vi "Grab Tag Information.vi"(8 "error in":errorcluster, 11 "VI Ref in":refnum<vi>) -> (0 "error out":errorcluster, 1 "Control Info":T1[](array[typedef]) {"tab level" items=["N/A", "FAB--icon--rounded", "outline--icon--rectangular", "outline--icon--rounded", "outline--text--rectangular", "outline--text--rounded", "nooutline--icon--rectangular", "nooutline--icon--rectangular--40x40", "nooutline--icon--rounded", "nooutline--text--rectangular", "nooutline--text--rounded", "tonal--icon--rectangular", "tonal--icon--rounded", "tonal--text--rectangular", "tonal--text--rounded", "filled--icon--rectangular", "filled--icon--rounded", "filled--text--rectangular", "filled--text--rounded"]; "Boolean Type" items=["N/A", "FAB--icon--rounded", "outline--icon--rectangular", "outline--icon--rounded", "outline--text--rectangular", "outline--text--rounded", "nooutline--icon--rectangular", "nooutline--icon--rectangular--40x40", "nooutline--icon--rounded", "nooutline--text--rectangular", "nooutline--text--rounded", "tonal--icon--rectangular", "tonal--icon--rounded", "tonal--text--rectangular", "tonal--text--rounded", "filled--icon--rectangular", "filled--icon--rounded", "filled--text--rectangular", "filled--text--rounded"]; "UI Theme Level" items=["N/A", "Primary", "Secondary", "Tertiary", "Error", "Primary Fixed", "Secondary Fixed", "Tertiary Fixed", "Label Only", "No Change"]}, 2 "map data":map{string, refnum<vi>}(c390), 3 "VI Ref out":refnum<vi>)   [LabVIEW 2021]
doc: "Get the tag data for all the controls on the front panel.\n\n<b>Code Developed By:</b>\nDaniel Coons\nTechnology Service Corporation\nwww.tsc.com/atcs"
uses:
  Material SubVIs/Material SubVIs.lvlib
  control info--typedef.ctl
  <vilib>/Utility/traverseref.llb/TRef TravTarget.ctl
  <vilib>/Utility/traverseref.llb/VI Scripting - Traverse.lvlib
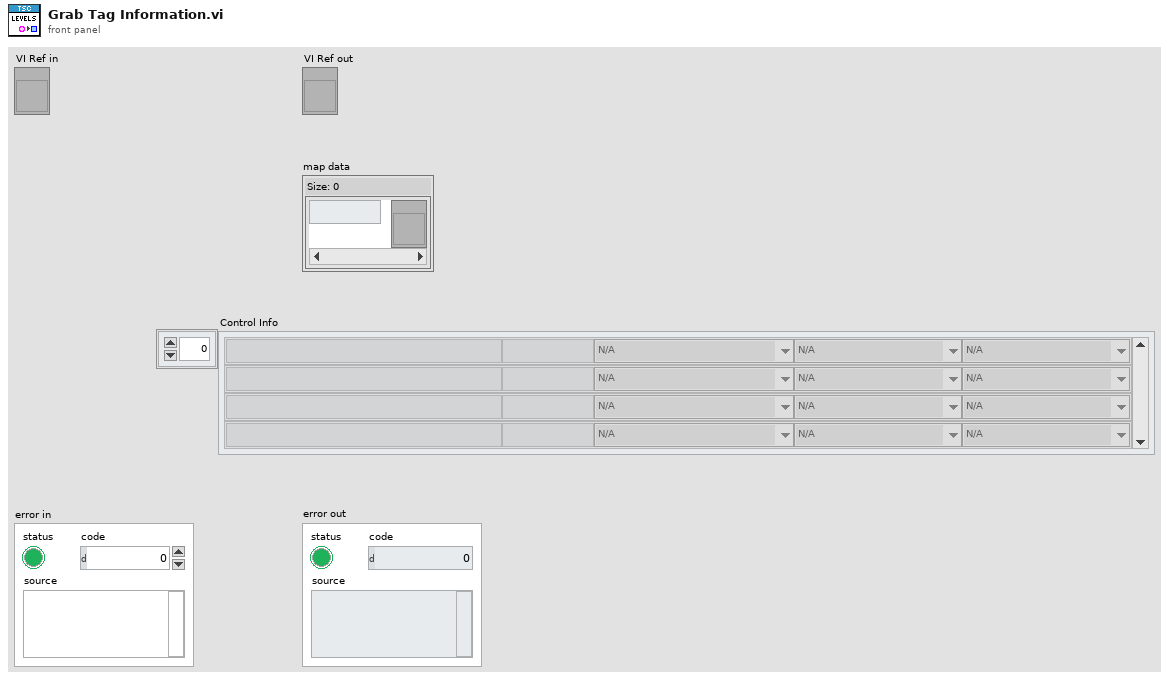
[diagram p1: front panel]
types:
  T1 = typedef "control info--typedef.ctl" = cluster{"label":string, "control type":string, "UI Theme Level":u16, "Boolean Type":u16, "tab level":u16}
  T2 = typedef "TRef TravTarget.ctl" = enum16{"FP", "BD", "Other"}
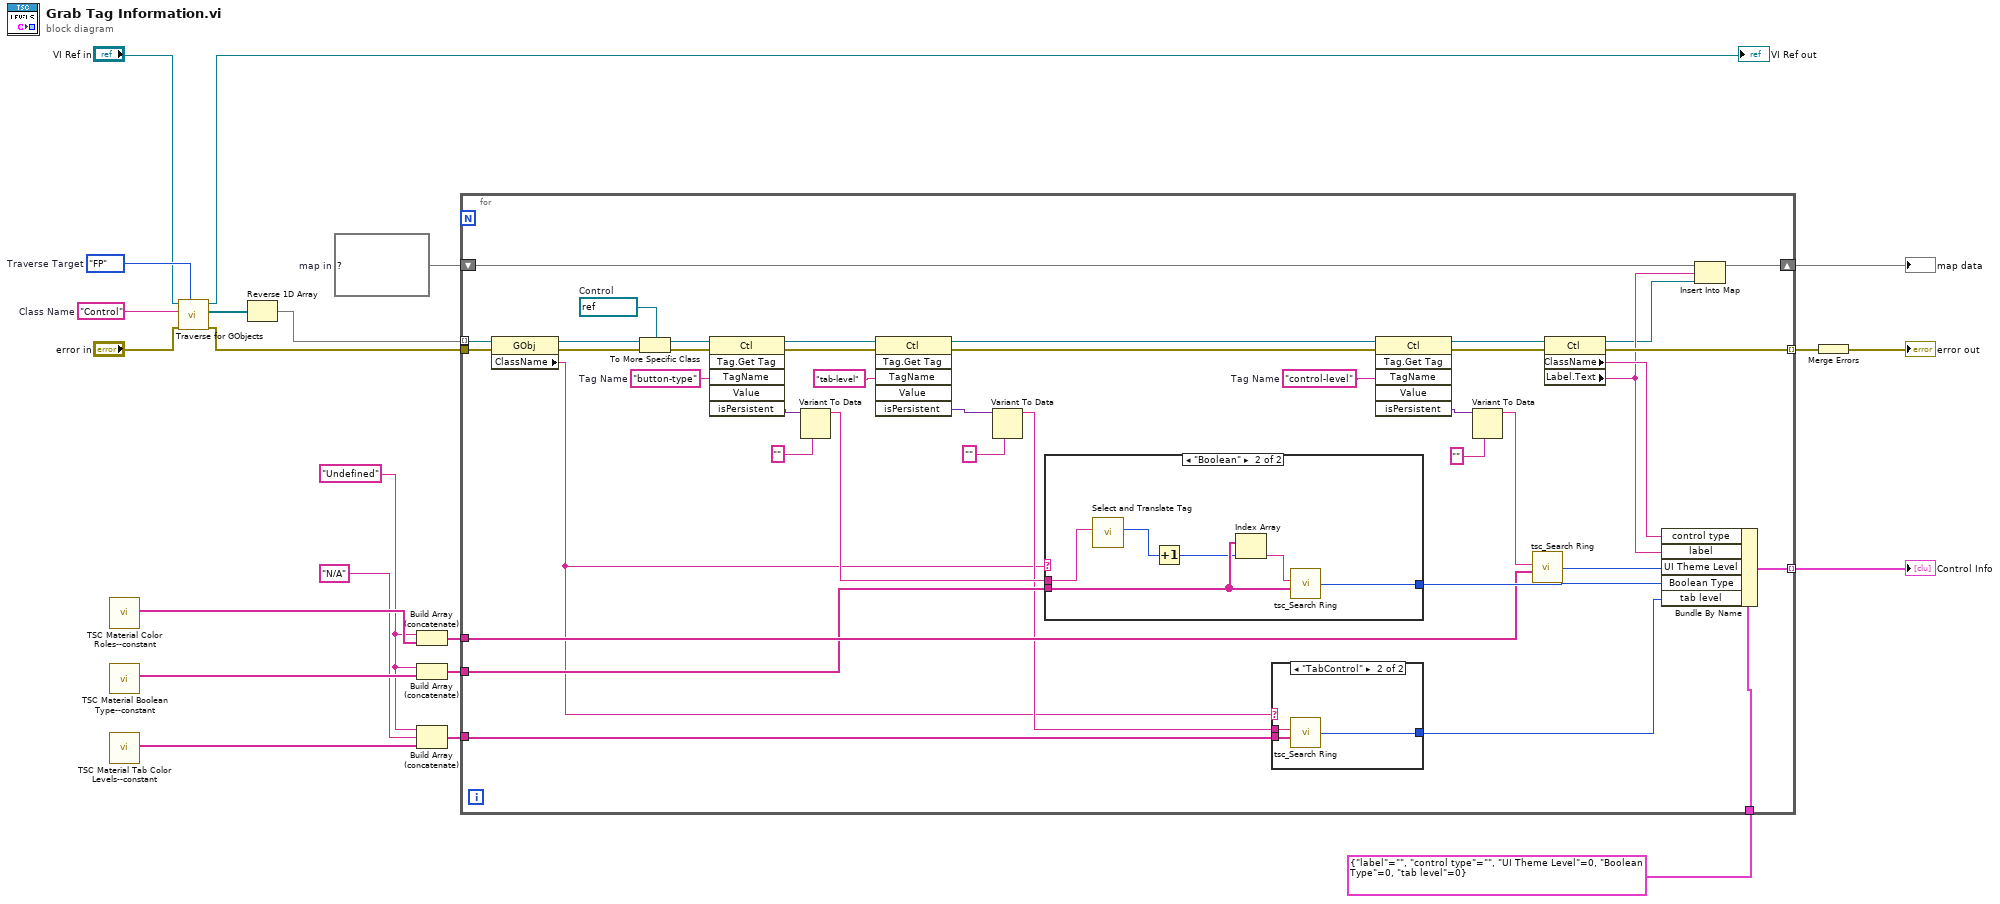
[diagram p0: block diagram]
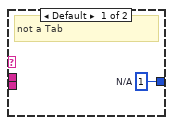
[diagram p2: hidden frame]
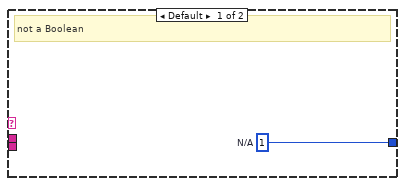
[diagram p3: hidden frame]
diagram:
  w11 = TRef_TravTarget."FP"  # Traverse Target
  w12 = "Control"  # Class Name
  w4 = "Undefined"
  w18 = map{string, refnum<vi>} {}  # map in
  n1 = call "TSC Material Color Roles--constant.vi"() -> ("Control Color Roles"=w15:string[])  [unwired: 11 in]
  n2 = call "TSC Material Boolean Type--constant.vi"() -> ("boolean types"=w5:string[])  [unwired: 11 in]
  n3 = call "TSC Material Tab Color Levels--constant.vi"() -> ("tab color levels"=w2:string[])  [unwired: 11 in]
  n4 = call <vilib>:"Traverse for GObjects.vi"("Traverse Target"=w11, "error in (no error)"="error in", "Class Name"=w12, "VI Refnum"="VI Ref in") -> ("error out"=w21:errorcluster, "References"=w10:refnum<vi>[], "dup VI Refnum"=→"VI Ref out":refnum<vi>)  [unwired: 4 in, 1 out]
  n5 = Reverse 1D Array(array=w10) -> (reversed array=w8:refnum<vi>[])
  n6 = Build Array (concatenate)(w4, w15) -> (w14:string[])
  n7 = Build Array (concatenate)(w4, w5) -> (w13:string[])
  n8 = Build Array (concatenate)(w4, "N/A", w2) -> (w1:string[])
  n9 = for {
    tunnel: w8 -> [w34] mode=indexing
    tunnel: w21 -> [w62]
    tunnel: [w59] -> w7 mode=indexing
    tunnel: T1 {"label"="", "control type"="", "UI Theme Level"=0, "Boolean Type"=0, "tab level"=0} ("control info") -> [w48]
    tunnel: [w46] -> w17 mode=indexing
    shift-right: [w44] -> w19
    shift-left: w18 -> [w45]
    tunnel: w14 -> [w37]
    tunnel: w13 -> [w36]
    tunnel: w1 -> [w24]
    w49 = refnum<vi> refnum  # Control
    w52 = "control-level"  # Tag Name
    w57 = "button-type"  # Tag Name
    n10 = property class="GObj"(reference=w34, error in=w62) -> (reference out=w33:refnum<vi>, error out=w35:errorcluster, "ClassName"=w25:string)
    n11 = To More Specific Class(target class=w49, reference=w33, error in=w35) -> (specific class reference=w50:refnum<vi>, error out=w58:errorcluster)
    n12 = invoke class="Ctl" method="Tag.Get Tag"(reference=w50, error in=w58, "TagName"=w57) -> (reference out=w31:refnum<vi>, error out=w61:errorcluster, "isPersistent"=w56:variant)  [unwired: 3 in, 3 out]
    n13 = Variant To Data(type="", Variant=w56) -> (data=w39:string)  [unwired: 1 in, 1 out]
    n14 = invoke class="Ctl" method="Tag.Get Tag"(reference=w31, error in=w61, "TagName"="tab-level" ("Tag Name")) -> (reference out=w30:refnum<vi>, error out=w32:errorcluster, "isPersistent"=w27:variant)  [unwired: 3 in, 3 out]
    n15 = Variant To Data(type="", Variant=w27) -> (data=w26:string)  [unwired: 1 in, 1 out]
    n16 = case shown="\"Boolean\"" w25 {
      tunnel: w39 -> [_ w72]
      tunnel: [w67 w73] -> w38
      tunnel: w36 -> [_ w70]
      frame Default {
        w67 = u16 1  # N/A
        # "not a Boolean"
      }
      frame "Boolean" {
        n17 = call "Select and Translate Tag.vi"("Current Item"=w72) -> ("index of element"=w71:i32)  [unwired: 10 in]
        n18 = Increment(x=w71) -> (x+1=w68:i32)
        n19 = Index Array(array=w70, index=w68) -> (element=w69:string)
        n20 = call "tsc_Search Ring.vi"("Values"=w70, "Search Item"=w69) -> ("Index"=w73:u16)  [unwired: 2 in]
      }
    }
    n21 = case shown="\"TabControl\"" w25 {
      tunnel: w26 -> [_ w66]
      tunnel: [w63 w65] -> w23
      tunnel: w24 -> [_ w64]
      frame Default {
        w63 = u16 1  # N/A
        # "not a Tab"
      }
      frame "TabControl" {
        n22 = call "tsc_Search Ring.vi"("Values"=w64, "Search Item"=w66) -> ("Index"=w65:u16)  [unwired: 2 in]
      }
    }
    n23 = invoke class="Ctl" method="Tag.Get Tag"(reference=w30, error in=w32, "TagName"=w52) -> (reference out=w51:refnum<vi>, error out=w60:errorcluster, "isPersistent"=w53:variant)  [unwired: 3 in, 3 out]
    n24 = Variant To Data(type="", Variant=w53) -> (data=w41:string)  [unwired: 1 in, 1 out]
    n25 = call "tsc_Search Ring.vi"("Values"=w37, "Search Item"=w41) -> ("Index"=w40:u16)  [unwired: 2 in]
    n26 = property class="Ctl"(reference=w51, error in=w60) -> (reference out=w42:refnum<vi>, error out=w59:errorcluster, "ClassName"=w47:string, "Label.Text"=w43:string)
    n27 = Bundle By Name(cluster=w48, "control type"=w47, "label"=w43, "UI Theme Level"=w40, "Boolean Type"=w38, "tab level"=w23) -> (w46:T1)
    n28 = Insert Into Map(map in=w45, key=w43, value=w42) -> (map out=w44:map{string, refnum<vi>})  [unwired: 2 out]
  }
  "map data" <- w19
  "Control Info" <- w17
  n29 = Merge Errors(w7) -> (→"error out":errorcluster)
